vi "QAB Actuators FPGA.vi"() -> ()   [LabVIEW 2019]
uses:
  <vilib>/Platform/TimedLoop/XDataNode/timing_clust.ctl
  <vilib>/Platform/TimedLoop/XDataNode/nitl_modes.ctl
  <vilib>/Platform/TimedLoop/XDataNode/wakeup.ctl
  <vilib>/rvi/Emulation/niFpgaGetClockAttributes.vi
  <vilib>/rvi/Emulation/niFpgaSctlEmulationGetInTimedLoop.vi
  <vilib>/rvi/Emulation/niFpgaEmulationReportErrorSimple.vi
  <vilib>/rvi/eio/common/nirviEmuTemplateMethod_errors.vi
  <vilib>/rvi/Emulation/niFpgaCriticalErrorInLSC.vi
  <vilib>/rvi/Emulation/niFpgaEmulationIsFPGAContextNoSignature.vi
  <vilib>/rvi/DataTransferAndStorage/Container/Common/niFpgaContainerGetUniqueNameForEmu.vi
  <vilib>/rvi/Memory/Memory_Emulation/niFpgaMemoryEmulationCacheClearOnFirstRun.vi
  <vilib>/rvi/Memory/Memory_Emulation/nirvimemoryEmulationManagerCache_MakeExclusive.vi
  <vilib>/rvi/Memory/Memory_Emulation/niFpgaMemoryEmulationValidateCache.vi
  <vilib>/rvi/Memory/Memory_Emulation/nirvimemoryEmulationManagerCache_InsertValue.vi
  <vilib>/Utility/error.llb/Clear Errors.vi
  <vilib>/rvi/Memory/Memory_Emulation/nirvimemoryEmulationManagerCache_ReleaseExclusive.vi
  <vilib>/rvi/Memory/Memory_Emulation/nirvimemoryEmulationManagerCache_GetValue.vi
  <vilib>/rvi/Memory/Memory_Emulation/nirvimemoryEmulationManagerCache_SetValue.vi
  <vilib>/rvi/Emulation/niFpgaProcessEmulError.vi
  <vilib>/rvi/DataTransferAndStorage/Container/Common/niFpgaContainerSetEmuInfo.vi
  <vilib>/rvi/eio/common/nirviEmuReportErrorAndStop.vi
  <vilib>/eio/EIONode/EIONode.xnode
  <vilib>/rvi/DataTransferAndStorage/Container/XNode/niFpgaContainer.xnode
  <vilib>/rvi/DataTransferAndStorage/Register/Emulation/niFpgaRegisterEmulation.vi
  <vilib>/Platform/TimedLoop/XDataNode/XDataNode.xnode
  <vilib>/rvi/LocalResourceManager/LocalResourceManager.xnode
  <vilib>/Platform/TimedLoop/XDataNode/XDNodeRunTimeDep.lvlib
panel:
  in  "Microstep Enable":bool
  in  "Microstep BD":sgl
  in  "Microstep AC":sgl
  out "BLDC Motor Tach Ticks":u32
  in  "DC Motor PWM Dir":bool
  in  "BLDC PWM (0-1)":sgl
  in  "Servo Period (1-2ms)":sgl
  out "DC Motor Tach Ticks":u32
  in  "Stepper Control 4":bool
  in  "Stepper Control 3":bool
  in  "Stepper Control 2":bool
  in  "Stepper Control 1":bool
  in  "LED Servo":bool
  in  "LED Stepper":bool
  in  "LED BLDC":bool
  in  "LED DC Motor":bool
  in  "LED Status":bool
  in  "DC Motor Linear Amplifier Enable":bool
  in  "DC Motor PWM (0-1)":sgl
  out "User Button":bool
  out "Power -15V":sgl
  out "Power +15V":sgl
  out "Power +5V":sgl
  out "Power +3.3V":sgl
  out "DC Motor Filtered Current":sgl
  in  "BLDC Drive Phase C":enum16{"H", "L", "Z"}(ring)
  in  "BLDC Drive Phase B":enum16{"H", "L", "Z"}(ring)
  in  "BLDC Drive Phase A":enum16{"H", "L", "Z"}(ring)
  in  "BLDC Encoder Reset":bool
  in  "BLDC Encoder Reset Value":i32
  out "BLDC Encoder Counter":i32
  out "BLDC Encoder RAW A/B/C":fxp<+,3,3> format="%02b"
  in  "LED3:0":fxp<+,4,4> format="%04b"
  in  "DC Linear Amplifier Value (+/-10)":sgl format="%#_17g"
  # "System"
  # "DC Motor"
  # "BLDC"
  # "Stepper"
  # "Servo"
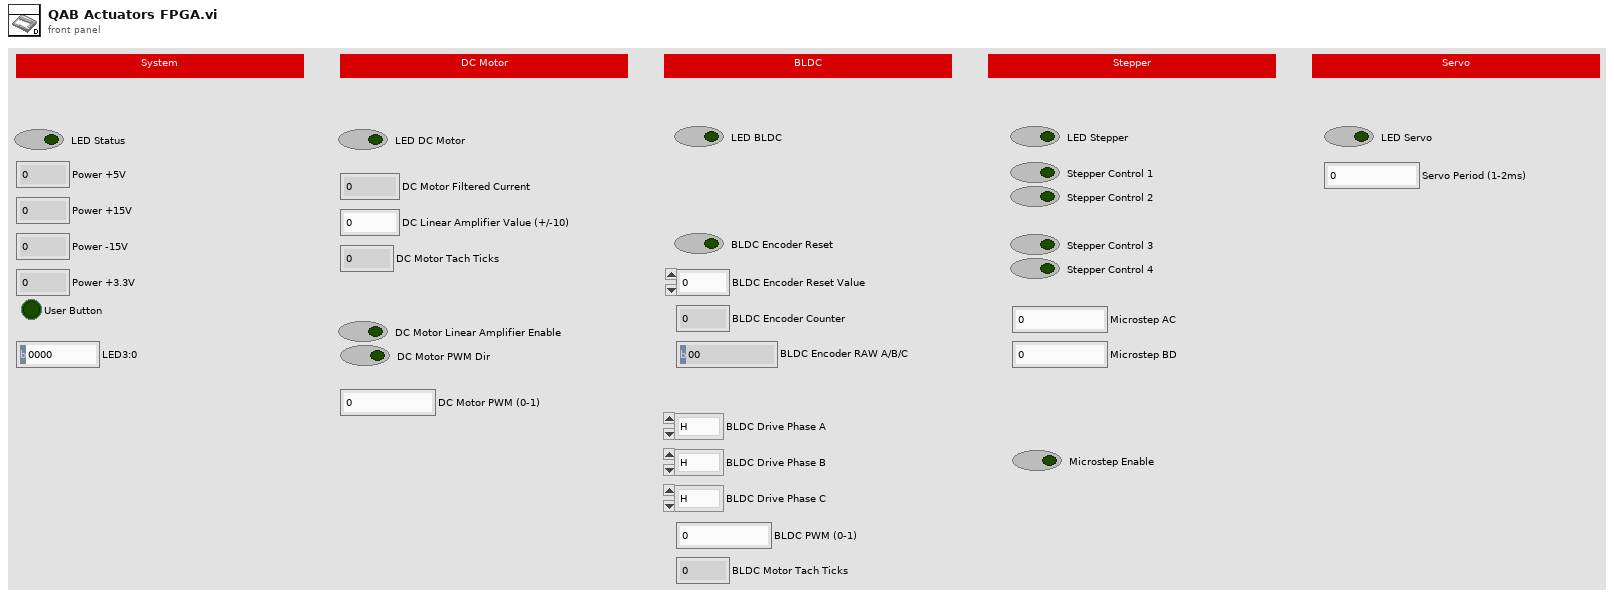
[diagram p1: front panel]
types:
  T1 = typedef "XDNodeRunTimeDep.lvlib/timing_clust.ctl" = cluster{"Expected End [f-1]":u64, "Actual End [f-1]":u64, "Finished Late? [f-1]":bool, "Expected End [i-1]":u64, "Actual End [i-1]":u64, "Finished Late? [i-1]":bool, "Expected Start [i]":u64, "Actual Start [i]":u64, "Expected Start [f]":u64, "Actual Start [f]":u64, "Source Name":string, "Structure Name":string, "Period":i64, "Deadline":i64, "Offset":i64, "Start":i64, "Priority":i32, "Timeout":i32, "Mode":T2, "Wakeup Reason":T3, "Error":errorcluster, "Source Type":string, "Secondary Source Type":string, "Global End Time":u64, "Global Start Time":u64, "Frame Duration":u64, "Iteration Duration":u64, "Assigned CPU":i32, "I/O Scan Engine Mode":u32}
  T2 = typedef "XDNodeRunTimeDep.lvlib/nitl_modes.ctl" = enum32{"No Change", "Process missed periods, maintain original phase", "Discard missed periods, maintain original phase", "Process missed periods, ignore original phase", "Discard missed periods, ignore original phase"}
  T3 = typedef "XDNodeRunTimeDep.lvlib/wakeup.ctl" = enum32{"Normal", "Aborted", "Asynchronous wakeup", "Timing source error", "Timed loop error", "Timeout"}
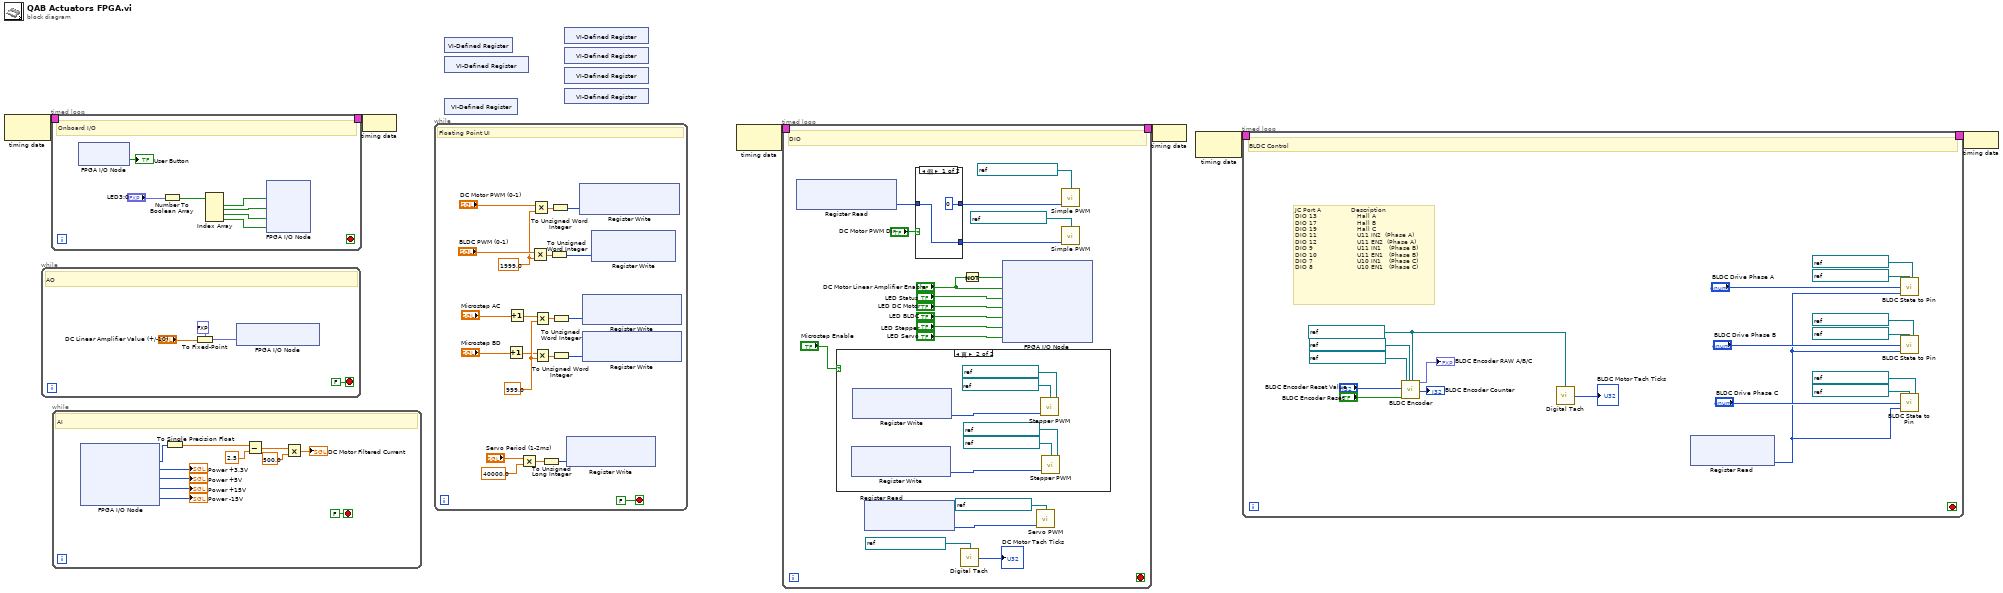
[diagram p0: block diagram]
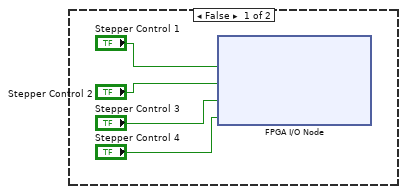
[diagram p2: hidden frame]
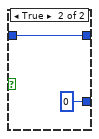
[diagram p3: hidden frame]
diagram:
  n1 = node-c288() -> (w6:T1)  [unwired: 1 in]
  n2 = while {
    stop <- FALSE stop-if-true
    # "AO"
    n3 = To Fixed-Point(fixed-point type=fxp<+/-,20,5> 0.0 ("ConnectorA/AO0"), number="DC Linear Amplifier Value (+/-10)") -> (fixed-point=w7:fxp<+/-,20,5>)
    n4 = xnode "FPGA I/O Node"("ConnectorA/AO0"=w7) -> ()  [unwired: 1 in, 1 out]
  }
  n5 = timed-loop {
    timing: w6 -> [_]
    timing-out: [_] -> w5
    stop <- _ stop-if-true
    # "Onboard I/O"
    n6 = xnode "FPGA I/O Node"() -> ("Button0"=→"User Button":bool)  [unwired: 1 in, 1 out]
    n7 = Number To Boolean Array(number="LED3:0") -> (Boolean array=w16:bool[])
    n8 = Index Array(array=w16) -> (element #1=w15:bool, element #2=w14:bool, element #3=w13:bool, element #4=w12:bool)  [unwired: 4 in]
    n9 = xnode "FPGA I/O Node"("LED0"=w15, "LED1"=w14, "LED2"=w13, "LED3"=w12) -> ()  [unwired: 4 in, 4 out]
  }
  n10 = while {
    stop <- FALSE stop-if-true
    # "AI"
    n11 = xnode "FPGA I/O Node"() -> ("ConnectorB/AI0"=w25:u16, "ConnectorA/AI3"=→"Power +3.3V":u16, "ConnectorA/AI2"=→"Power +5V":u16, "ConnectorA/AI1"=→"Power +15V":u16, "ConnectorA/AI0"=→"Power -15V":u16)  [unwired: 5 in, 5 out]
    n12 = To Single Precision Float(number=w25) -> (single precision float=w20:sgl)
    n13 = Subtract(x=w20, y=sgl 2.5) -> (x-y=w23:sgl)
    n14 = Multiply(x=w23, y=sgl 500.0) -> (x*y=→"DC Motor Filtered Current":sgl)
  }
  n15 = node-c288(w5) -> ()
  n16 = while {
    stop <- FALSE stop-if-true
    w35 = sgl 999.0 ("y")
    w36 = sgl 1999.0 ("y")
    # "Floating Point UI"
    n17 = Increment(x="Microstep BD") -> (x+1=w31:sgl)
    n18 = Increment(x="Microstep AC") -> (x+1=w33:sgl)
    n19 = Multiply(x="Servo Period (1-2ms)", y=sgl 40000.0) -> (x*y=w49:sgl)
    n20 = Multiply(x="BLDC PWM (0-1)", y=w36) -> (x*y=w43:sgl)
    n21 = Multiply(x="DC Motor PWM (0-1)", y=w36) -> (x*y=w48:sgl)
    n22 = Multiply(x=w33, y=w35) -> (x*y=w40:sgl)
    n23 = Multiply(x=w31, y=w35) -> (x*y=w39:sgl)
    n24 = To Unsigned Long Integer(number=w49) -> (unsigned 32bit integer=w44:u32)
    n25 = To Unsigned Word Integer(number=w43) -> (unsigned 16bit integer=w41:u16)
    n26 = To Unsigned Word Integer(number=w48) -> (unsigned 16bit integer=w45:u16)
    n27 = To Unsigned Word Integer(number=w40) -> (unsigned 16bit integer=w38:u16)
    n28 = To Unsigned Word Integer(number=w39) -> (unsigned 16bit integer=w37:u16)
    n29 = xnode ("Register Write")("数据"=w44) -> ()  [unwired: 1 in, 1 out]
    n30 = xnode ("Register Write")("数据"=w45) -> ()  [unwired: 1 in, 1 out]
    n31 = xnode ("Register Write")("数据"=w38) -> ()  [unwired: 1 in, 1 out]
    n32 = xnode ("Register Write")("数据"=w37) -> ()  [unwired: 1 in, 1 out]
    n33 = xnode ("Register Write")("数据"=w41) -> ()  [unwired: 1 in, 1 out]
  }
  n34 = xnode "VI-Defined Register"() -> ()  [unwired: 1 out]
  n35 = xnode "VI-Defined Register"() -> ()  [unwired: 1 out]
  n36 = xnode "VI-Defined Register"() -> ()  [unwired: 1 out]
  n37 = xnode "VI-Defined Register"() -> ()  [unwired: 1 out]
  n38 = xnode "VI-Defined Register"() -> ()  [unwired: 1 out]
  n39 = xnode "VI-Defined Register"() -> ()  [unwired: 1 out]
  n40 = xnode "VI-Defined Register"() -> ()  [unwired: 1 out]
  n41 = node-c288() -> (w2:T1)  [unwired: 1 in]
  n42 = timed-loop {
    timing: w2 -> [_]
    timing-out: [_] -> w1
    stop <- _ stop-if-true
    # "DIO"
    n43 = xnode ("Register Read")() -> ("数据"=w55:u16)  [unwired: 1 in, 1 out]
    n44 = case shown="真" "Microstep Enable" {
      frame False {
        n45 = xnode "FPGA I/O Node"("ConnectorB/DIO5"="Stepper Control 1", "ConnectorB/DIO9"="Stepper Control 2", "ConnectorB/DIO7"="Stepper Control 3", "ConnectorB/DIO11"="Stepper Control 4") -> ()  [unwired: 4 in, 4 out]
      }
      frame True {
        n46 = xnode ("Register Write")() -> ("数据"=w74:u16)  [unwired: 1 in, 1 out]
        n47 = xnode ("Register Write")() -> ("数据"=w77:u16)  [unwired: 1 in, 1 out]
        n48 = call "Stepper PWM.vi"("Drive Pin 2"=refnum<k21> "ConnectorC/DIO6" ("Drive Pin"), "Drive Pin 1"=refnum<k21> "ConnectorB/DIO3" ("Drive Pin"), "Duty Cycle (0-1999)"=w77) -> ()  [unwired: 2 in]
        n49 = call "Stepper PWM.vi"("Drive Pin 2"=refnum<k21> "ConnectorB/DIO4" ("Drive Pin"), "Drive Pin 1"=refnum<k21> "ConnectorA/DIO1" ("Drive Pin"), "Duty Cycle (0-1999)"=w74) -> ()  [unwired: 2 in]
      }
    }
    n50 = xnode ("Register Read")() -> ("数据"=w57:u32)  [unwired: 1 in, 1 out]
    n51 = case shown="假" "DC Motor PWM Dir" {
      tunnel: w55 -> [w81 w83]
      tunnel: [u16 0 ("Data") w83] -> w54
      tunnel: [w81 u16 0 ("Data")] -> w53
      frame False {
      }
      frame True {
      }
    }
    n52 = call "Digital Tach.vi"("Input Pin"=refnum<k21> "ConnectorA/DIO10" ("Drive Pin")) -> ("Tach Ticks"=→"DC Motor Tach Ticks":u32)  [unwired: 3 in]
    n53 = Not(x="DC Motor Linear Amplifier Enable") -> (.not. x?=w59:bool)
    n54 = xnode "FPGA I/O Node"("ConnectorA/DIO14"=w59, "ConnectorA/DIO15"="DC Motor Linear Amplifier Enable", "ConnectorB/DIO0"="LED Status", "ConnectorA/DIO1"="LED DC Motor", "ConnectorB/DIO8"="LED BLDC", "ConnectorB/DIO9"="LED Stepper", "ConnectorC/DIO7"="LED Servo") -> ()  [unwired: 7 in, 7 out]
    n55 = call "Servo PWM.vi"("Drive Pin"=refnum<k21> "ConnectorC/DIO2", "Duty Cycle"=w57) -> ()  [unwired: 3 in]
    n56 = call "Simple PWM.vi"("Drive Pin"=refnum<k21> "ConnectorA/DIO13", "Duty Cycle (0-1999)"=w54) -> ()  [unwired: 3 in]
    n57 = call "Simple PWM.vi"("Drive Pin"=refnum<k21> "ConnectorA/DIO9", "Duty Cycle (0-1999)"=w53) -> ()  [unwired: 3 in]
  }
  n58 = node-c288(w1) -> ()
  n59 = node-c288() -> (w4:T1)  [unwired: 1 in]
  n60 = timed-loop {
    timing: w4 -> [_]
    timing-out: [_] -> w3
    stop <- _ stop-if-true
    w86 = refnum<k21> "ConnectorC/DIO1" ("C")
    # "JC Port A               Description\nDIO 13\t\t                  Hall A\nDIO 17\t\t                  Hall B\nDIO 19\t\t                  Hall C\nDIO 11\t\t                  U11 IN2  (Phase A)\nDIO 12\t\t                  U11 EN2  (Phase A)\nDIO 9\t\t                   \tU11 IN1    (Phase B)\nDIO 10\t\t                  U11 EN1   (Phase B)\nDIO 7\t\t                    U10 IN1    (Phase C)\nDIO 8\t\t                    U10 EN1   (Phase C)"
    # "BLDC Control"
    n61 = call "BLDC Encoder.vi"("Encoder Reset Value"="BLDC Encoder Reset Value", "Encoder Reset"="BLDC Encoder Reset", "A"=refnum<k21> "ConnectorA/DIO8" ("B"), "B"=refnum<k21> "ConnectorC/DIO3" ("A"), "C"=w86) -> ("Encoder RAW A/B/C"=→"BLDC Encoder RAW A/B/C":fxp<+,3,3>, "Encoder Counter"=→"BLDC Encoder Counter":i32)  [unwired: 12 in, 1 out]
    n62 = call "Digital Tach.vi"("Input Pin"=w86) -> ("Tach Ticks"=→"BLDC Motor Tach Ticks":u32)  [unwired: 3 in]
    n63 = xnode ("Register Read")() -> ("数据"=w88:u16)  [unwired: 1 in, 1 out]
    n64 = call "BLDC State to Pin.vi"("Enable"=refnum<k21> "ConnectorA/DIO7", "Drive Pin"=refnum<k21> "ConnectorA/DIO6", "Compare Value"=w88, "State"="BLDC Drive Phase A") -> ()  [unwired: 1 in]
    n65 = call "BLDC State to Pin.vi"("Enable"=refnum<k21> "ConnectorA/DIO5", "Drive Pin"=refnum<k21> "ConnectorA/DIO4", "Compare Value"=w88, "State"="BLDC Drive Phase B") -> ()  [unwired: 1 in]
    n66 = call "BLDC State to Pin.vi"("Enable"=refnum<k21> "ConnectorA/DIO3", "Drive Pin"=refnum<k21> "ConnectorA/DIO2", "Compare Value"=w88, "State"="BLDC Drive Phase C") -> ()  [unwired: 1 in]
  }
  n67 = node-c288(w3) -> ()
